vi "New Verify.vi"(11 "LUnit Test Case In":refnum<class "Test Case.lvclass">) -> (0 "error out":errorcluster, 3 "LUnit Test Case Out":refnum<class "Test Case.lvclass">)   [LabVIEW 2020, in "LUnit.Extension.lvlib"]
uses:
  LUnit.Extension.lvlib
  <vilib>/Astemes/LUnit/Test Case.lvclass
  Approval Tests/Options/Options.lvclass/Options.ctl
  Approval Tests/Naming Data/Naming Data.lvclass/Naming Data.ctl
  <vilib>/Astemes/LUnit/Test Case.lvclass/Test Case.ctl
  535bad47-a2ae-4fd4-bb72-03c2d2b06672.vi
  535bad47-a2ae-4fd4-bb72-03c2d2b06672.vi/1e051690-6811-4db0-8b8f-f6ad9423d026.vi
  Approval Tests/Replace if Empty.vi
  <vilib>/Astemes/LUnit/Palette/Pass If.vi
  Approval Tests/Options/Update Test Name if Not Defined.vi
  Approval Tests/Verify Core.vi
  535bad47-a2ae-4fd4-bb72-03c2d2b06672.vi/1e051690-6811-4db0-8b8f-f6ad9423d026.vi/93c5622b-9fb7-41e0-8c76-3fde37e94e34.vi
  Approval Tests/Options/Read Scrubber.vi
  <vilib>/Astemes/LUnit/Core/LUnit Test Case/Private/Append Fail Result.vi
  <vilib>/Astemes/LUnit/Core/LUnit Test Case/Private/Append Pass Result.vi
  Approval Tests/Naming Data/Read Test VI Name.vi
  Approval Tests/Naming Data/Write Test VI Name.vi
  Approval Tests/Options/Read Namer.vi
  Approval Tests/Options/Read Naming Data.vi
  Approval Tests/Options/Read Reporter.vi
  Approval Tests/Options/Read Text Comparator.vi
  535bad47-a2ae-4fd4-bb72-03c2d2b06672.vi/1e051690-6811-4db0-8b8f-f6ad9423d026.vi/93c5622b-9fb7-41e0-8c76-3fde37e94e34.vi/04cb982b-2eda-40d0-8d7e-90f8e0b569b2.vi
  <vilib>/Astemes/LUnit/Core/LUnit Test Case/Private/Run In UI.vi
  <vilib>/Utility/error.llb/Clear Errors.vi
  Approval Tests/Options/Add Label to Namer.vi
  Approval Tests/conv EOL.vi
  <vilib>/Utility/libraryn.llb/Check if File or Folder Exists.vi
  Approval Tests/Reporter/Report.vi
  Approval Tests/Options/Options.lvclass
  Approval Tests/Scrubber/Scrubber.lvclass
  Approval Tests/Namer/Namer.lvclass
  Approval Tests/Naming Data/Naming Data.lvclass
  Approval Tests/Reporter/Reporter.lvclass
  Approval Tests/Text Comparator/Text Comparator.lvclass
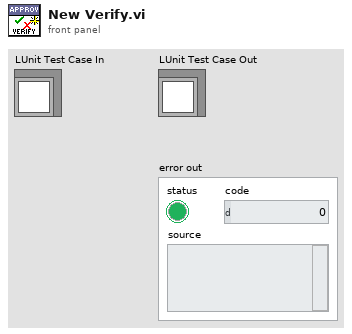
[diagram p1: front panel]
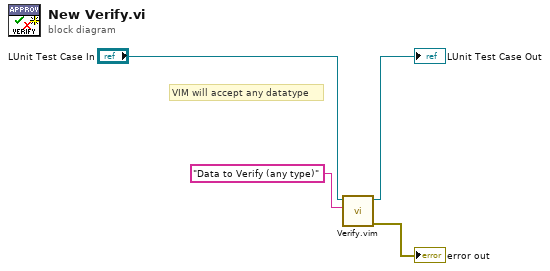
[diagram p0: block diagram]
diagram:
  # "VIM will accept any datatype"
  n1 = call "Verify.vim"("Test Data"="Data to Verify (any type)", "LUnit Test Case In"="LUnit Test Case In") -> ("error out"=→"error out":errorcluster, "LUnit Test Case Out"=→"LUnit Test Case Out":refnum<class "Test Case.lvclass">)  [unwired: 8 in]
